vi "Get SLSC Product Name.vi"(8 "error in (no error)":errorcluster, 11 "SLSC Module Resource":refnum<k21>) -> (0 "error out":errorcluster, 3 "Dev.ProductName":string)   [LabVIEW 2017, in "NI-SWITCH System Explorer.lvlib"]
uses:
  NI-SWITCH System Explorer.lvlib
  <vilib>/SLSC/Initialize Session with Devices.vi
  <vilib>/SLSC/Close Session.vi
  <vilib>/SLSC/SLSC.lvlib
  <resource>/objmgr/slsc.rc
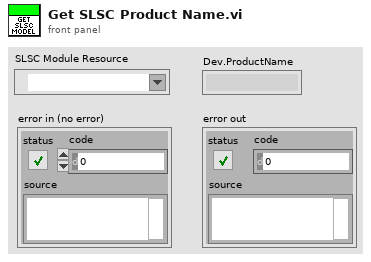
[diagram p1: front panel]
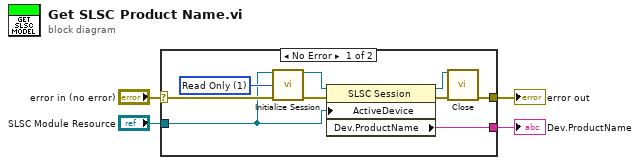
[diagram p0: block diagram]
diagram:
  n1 = case shown="No Error" "error in (no error)" {
    selector: "error in (no error)" -> [w7 w14]
    tunnel: [w6 _] -> w4
    tunnel: [w13 w14] -> w3
    tunnel: "SLSC Module Resource" -> [w5 _]
    frame No Error {
      w8 = 1 items=["None"=0, "Read Only"=1, "Read/Write"=3] ("reservation access (Read/Write)")
      n2 = call-poly <vilib>:"Initialize Session.vi"("devices"=w5, "reservation access (Read/Write)"=w8, "error in (no error)"=w7) -> ("session out"=w9:refnum<k21>, "error out"=w10:errorcluster)  [unwired: 11 in]
      n3 = property class="SLSC Session"(reference=w9, error in=w10, "ActiveDevice"=w5) -> (reference out=w12:refnum<k21>, error out=w11:errorcluster, "Dev.ProductName"=w6:string)
      n4 = call-poly <vilib>:"Close.vi"("session in"=w12, "error in (no error)"=w11) -> ("error out"=w13:errorcluster)  [unwired: 13 in]
    }
    frame Error {
    }
  }
  "Dev.ProductName" <- w4
  "error out" <- w3
